vi "SERIAL_Open.vi"(7 "Serial Port (MXP)":T1=enum."MXP TTL", 9 "Reconnect":bool, 10 "Update Rate (4Hz-60Hz)":u8=50, 11 "Nav6Mode (ProcessedData)":T2) -> (0 "error out":errorcluster, 1 "Opened":bool, 3 "navX Ref":T3={"SerialPortRef"={"DevStatus"={"status"=FALSE, "code"=0, "source"=""}, "Serial Port Name"=""}, "Board Information"={"WhoAmI (50 | 0x32)"=0, "Board Revision"=0, "Firmware Major Version"=0, "Firmware Minor Version"=0, "NAVX_BOARD_CAPABILITY"={"OMNIMOUNT"=FALSE, "YAW_RESET"=FALSE, "VEL_AND_DISP"=FALSE}, "NAVX_BOARD_YAW_AXIS"={"BOARD_YAW_AXIS_UP"=FALSE, "BOARD_YAW_AXIS"=0}}, "Status"={"Update Rate Hz"=0, "Accelerometer Full-Scale Range"=0, "Gyro Full-Scale Range"=0, "NAVX_OP_STATUS"=0, "NAVX_CAL_STATUS"=0, "NAVX_SELFTEST_STATUS"=0, "NAVX_SENSOR_STATUS"={"MOVING"=FALSE, "YAW_STABLE"=FALSE, "MAG_DISTURBANCE"=FALSE, "ALTITUDE_VALID"=FALSE, "SEALEVEL_PRESS_SET"=FALSE, "FUSED_HEADING_VALID"=FALSE}}, "Offsets"={"Yaw"=0.0, "Quat W"=0.0, "Quat X"=0.0, "Quat Y"=0.0, "Quat Z"=0.0}, "Update Rate (4Hz-60Hz)"=50, "Nav6Mode (YPR)"=enum."RawSensorData", "refnum name"="", "error"={"status"=FALSE, "code"=0, "source"=""}, "Loop VI Refnum"=refnum, "Serial Port"=enum."Onboard RS-232"} {"Status"."NAVX_OP_STATUS" items=["INITIALIZING", "SELFTEST_IN_PROGRESS", "ERROR", "IMU_AUTOCAL_IN_PROGRESS", "NORMAL"]; "Status"."NAVX_CAL_STATUS" items=["IMU_CAL_STATE_MASK"=3, "IMU_CAL_INPROGRESS"=0, "IMU_CAL_ACCUMULATE"=1, "IMU_CAL_COMPLETE"=2, "MAG_CAL_COMPLETE"=4, "BARO_CAL_COMPLETE"=8]})   [LabVIEW 2014, in "navX-MXP IMU.lvlib"]
uses:
  navX-MXP IMU.lvlib
  TypeDefs/navX Serial DevRef.ctl
  <vilib>/Rock Robotics/WPI/SerialPort/WPI_SerialPortRef.ctl
  COMMON/TypeDefs/Data TypeDefs/navX Board Information.ctl
  COMMON/TypeDefs/Value TypeDefs/navX NAVX_BOARD_CAPABILITY.ctl
  COMMON/TypeDefs/Value TypeDefs/navX NAVX_BOARD_YAW_AXIS.ctl
  COMMON/TypeDefs/Data TypeDefs/navX Status Data.ctl
  COMMON/TypeDefs/Value TypeDefs/navX NAVX_OP_STATUS.ctl
  COMMON/TypeDefs/Value TypeDefs/navX NAVX_CAL_STATUS.ctl
  COMMON/TypeDefs/Value TypeDefs/navX NAVX_SENSOR_STATUS.ctl
  TypeDefs/navX Serial Mode.ctl
  NI WPI/WPI_SerialPort_USB.ctl
  <vilib>/Rock Robotics/SystemInterfaces/Utilities/FPGA_UtilitiesRead LocalTime.vi
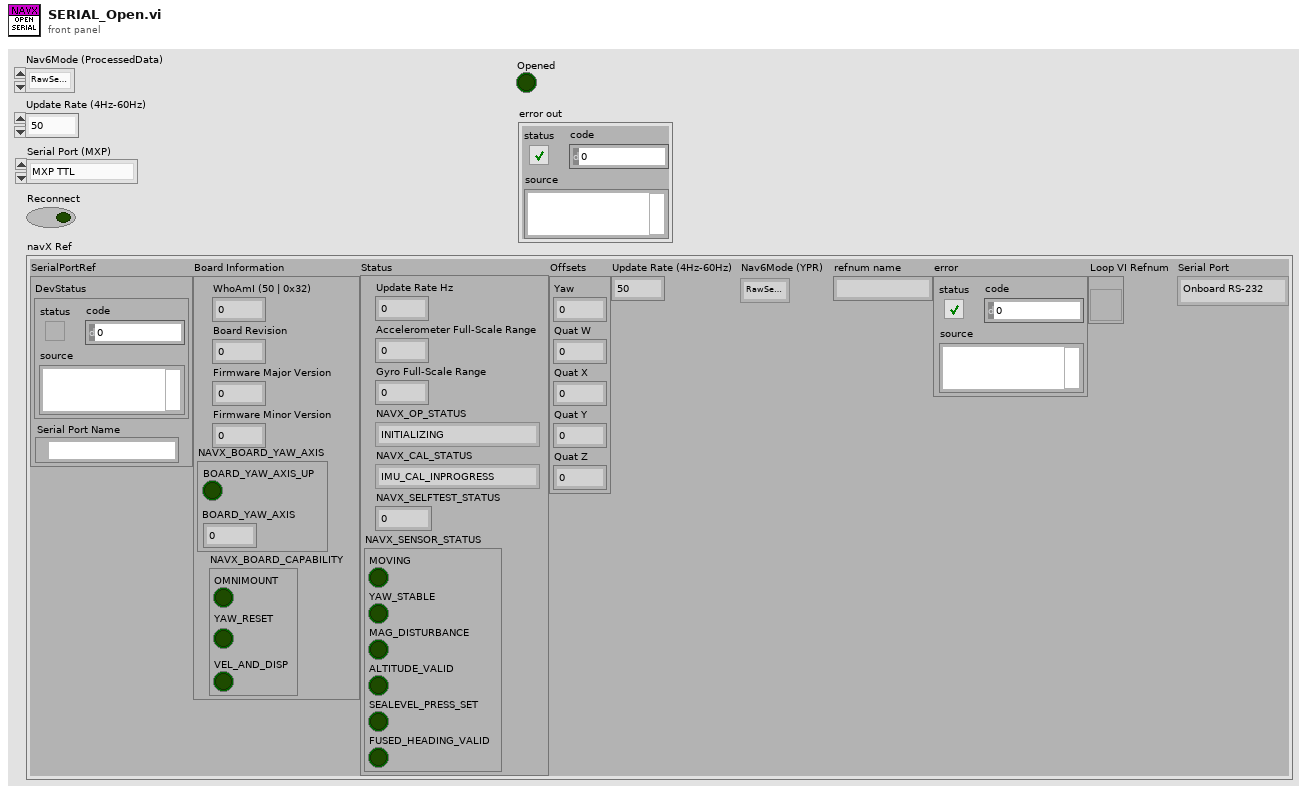
[diagram p1: front panel]
types:
  T1 = typedef "navX-MXP IMU.lvlib/WPI_SerialPort_USB.ctl" = enum16{"Onboard RS-232", "MXP TTL", "USB"}
  T2 = typedef "navX-MXP IMU.lvlib/navX Serial Mode.ctl" = enum16{"RawSensorData", "ProcessedData"}
  T3 = typedef "navX-MXP IMU.lvlib/navX Serial DevRef.ctl" = cluster{"SerialPortRef":T4, "Board Information":T5, "Status":T8, "Offsets":cluster{"Yaw":dbl, "Quat W":dbl, "Quat X":dbl, "Quat Y":dbl, "Quat Z":dbl}, "Update Rate (4Hz-60Hz)":u8, "Nav6Mode (YPR)":T2, "refnum name":string, "error":errorcluster, "Loop VI Refnum":refnum<vi>, "Serial Port":T1}
  T4 = typedef "WPI_SerialPortRef.ctl" = cluster{"DevStatus":errorcluster, "Serial Port Name":refnum<visa-resource-name>}
  T5 = typedef "navX-MXP IMU.lvlib/navX Board Information.ctl" = cluster{"WhoAmI (50 | 0x32)":u8, "Board Revision":u8, "Firmware Major Version":u8, "Firmware Minor Version":u8, "NAVX_BOARD_CAPABILITY":T6, "NAVX_BOARD_YAW_AXIS":T7}
  T6 = typedef "navX-MXP IMU.lvlib/navX NAVX_BOARD_CAPABILITY.ctl" = cluster{"OMNIMOUNT":bool, "YAW_RESET":bool, "VEL_AND_DISP":bool}
  T7 = typedef "navX-MXP IMU.lvlib/navX NAVX_BOARD_YAW_AXIS.ctl" = cluster{"BOARD_YAW_AXIS_UP":bool, "BOARD_YAW_AXIS":u8}
  T8 = typedef "navX-MXP IMU.lvlib/navX Status Data.ctl" = cluster{"Update Rate Hz":u8, "Accelerometer Full-Scale Range":u8, "Gyro Full-Scale Range":u16, "NAVX_OP_STATUS":T9, "NAVX_CAL_STATUS":T10, "NAVX_SELFTEST_STATUS":u8, "NAVX_SENSOR_STATUS":T11}
  T9 = typedef "navX-MXP IMU.lvlib/navX NAVX_OP_STATUS.ctl" = u8
  T10 = typedef "navX-MXP IMU.lvlib/navX NAVX_CAL_STATUS.ctl" = u8
  T11 = typedef "navX-MXP IMU.lvlib/navX NAVX_SENSOR_STATUS.ctl" = cluster{"MOVING":bool, "YAW_STABLE":bool, "MAG_DISTURBANCE":bool, "ALTITUDE_VALID":bool, "SEALEVEL_PRESS_SET":bool, "FUSED_HEADING_VALID":bool}
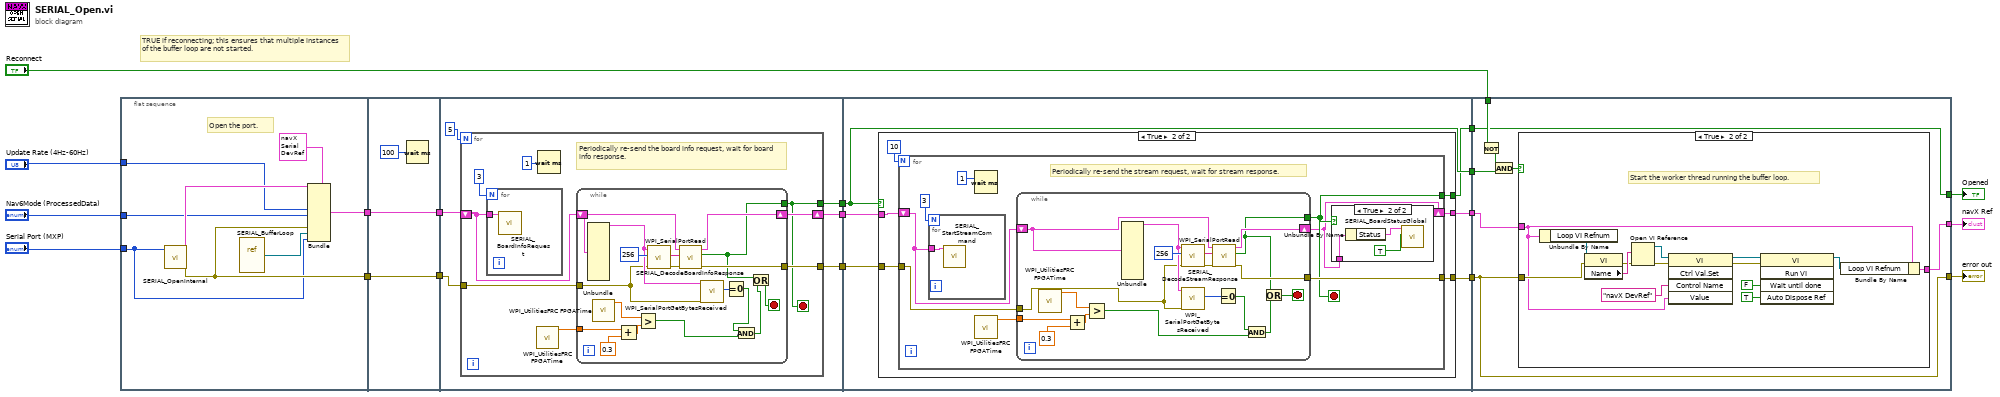
[diagram p0: block diagram]
diagram:
  # "TRUE if reconnecting; this ensures that multiple instances of the buffer loop are not started."
  n1 = flat-sequence {
    tunnel: [w26] -> w18
    tunnel: [w22] -> w7
    tunnel: "Update Rate (4Hz-60Hz)" -> [w21]
    tunnel: "Nav6Mode (ProcessedData)" -> [w20]
    tunnel: "Serial Port (MXP)" -> [w19]
    tunnel: w18 -> [w27]
    tunnel: [w28] -> w8
    tunnel: w7 -> [w28]
    tunnel: [w27] -> w6
    tunnel: [w30] -> w15
    tunnel: [w35] -> w12
    tunnel: [w34] -> w10
    tunnel: w8 -> [w31]
    tunnel: w6 -> [w33]
    tunnel: w15 -> [w64]
    tunnel: [w63] -> w14
    tunnel: [w67] -> w13
    tunnel: w12 -> [w66]
    tunnel: [w65] -> w11
    tunnel: w10 -> [w68]
    tunnel: [w68] -> w9
    tunnel: [w108] -> w1
    tunnel: [w115] -> w17
    tunnel: [w114] -> w16
    tunnel: w14 -> [w115]
    tunnel: w13 -> [w108]
    tunnel: w11 -> [w113]
    tunnel: w9 -> [w112]
    tunnel: "Reconnect" -> [w111]
    frame #0 {
      # "Open the port."
      n2 = call "SERIAL_OpenInternal.vi"("Serial Port (MXP)"=w19) -> ("error out"=w22:errorcluster, "SerialPortRef"=w23:T4)  [unwired: 8 in, 1 out]
      n3 = vi-ref "SERIAL_BufferLoop.vi"() -> (w25:refnum<vi>)
      n4 = Bundle(cluster=T3 {"SerialPortRef"={"DevStatus"={"status"=FALSE, "code"=0, "source"=""}, "Serial Port Name"=""}, "Board Information"={"WhoAmI (50 | 0x32)"=0, "Board Revision"=0, "Firmware Major Version"=0, "Firmware Minor Version"=0, "NAVX_BOARD_CAPABILITY"={"OMNIMOUNT"=FALSE, "YAW_RESET"=FALSE, "VEL_AND_DISP"=FALSE}, "NAVX_BOARD_YAW_AXIS"={"BOARD_YAW_AXIS_UP"=FALSE, "BOARD_YAW_AXIS"=0}}, "Status"={"Update Rate Hz"=0, "Accelerometer Full-Scale Range"=0, "Gyro Full-Scale Range"=0, "NAVX_OP_STATUS"=0, "NAVX_CAL_STATUS"=0, "NAVX_SELFTEST_STATUS"=0, "NAVX_SENSOR_STATUS"={"MOVING"=FALSE, "YAW_STABLE"=FALSE, "MAG_DISTURBANCE"=FALSE, "ALTITUDE_VALID"=FALSE, "SEALEVEL_PRESS_SET"=FALSE, "FUSED_HEADING_VALID"=FALSE}}, "Offsets"={"Yaw"=0.0, "Quat W"=0.0, "Quat X"=0.0, "Quat Y"=0.0, "Quat Z"=0.0}, "Update Rate (4Hz-60Hz)"=50, "Nav6Mode (YPR)"=enum."RawSensorData", "refnum name"="", "error"={"status"=FALSE, "code"=0, "source"=""}, "Loop VI Refnum"=refnum, "Serial Port"=enum."Onboard RS-232"} ("navX Ref Object"), "SerialPortRef"=w23, "Update Rate (4Hz-60Hz)"=w21, "Nav6Mode (YPR)"=w20, "error"=w22, "Loop VI Refnum"=w25, "Serial Port"=w19) -> (w26:T3)  [unwired: 4 in]
    }
    frame #1 {
      n5 = Wait (ms)(milliseconds to wait=u32 100) -> ()  [unwired: 1 out]
    }
    frame #2 {
      n6 = for {
        N: 5 -> [_]
        tunnel: [w42] -> w30
        tunnel: [w41] -> w34
        shift-right: [w43] -> w35
        shift-left: w33 -> [w39]
        tunnel: w31 -> [w38]
        stop <- w41 stop-if-true
        # "Periodically re-send the board info request, wait for board info response."
        n7 = for {
          N: 3 -> [_]
          tunnel: w39 -> [w44]
          n8 = call "SERIAL_BoardInfoRequest.vi"("navX Ref"=w44) -> ()  [unwired: 10 in, 1 out]
        }
        n9 = call <vilib>:"WPI_UtilitiesFRC FPGATime.vi"() -> ("FPGA Time"=w37:dbl)  [unwired: 10 in, 1 out]
        n10 = Wait (ms)(milliseconds to wait=u32 1) -> ()  [unwired: 1 out]
        n11 = while {
          tunnel: [w61] -> w42
          tunnel: [w55] -> w41
          shift-right: [w62] -> w43
          shift-left: w39 -> [w60]
          tunnel: w38 -> [w53]
          tunnel: w37 -> [w49]
          stop <- w54 stop-if-true
          n12 = Unbundle(w60) -> ("SerialPortRef"=w56:T4)  [unwired: 9 out]
          n13 = call <vilib>:"WPI_UtilitiesFRC FPGATime.vi"() -> ("FPGA Time"=w52:dbl)  [unwired: 10 in, 1 out]
          n14 = Add(x=w49, y=0.3) -> (x+y=w51:dbl)
          n15 = Greater?(x=w52, y=w51) -> (0:w48:bool)
          n16 = call <vilib>:"WPI_SerialPortRead.vi"("error in (no error)"=w53, "Num Bytes to Read"=u32 256, "SerialPortRef"=w56) -> ("error out"=w58:errorcluster, "Buffer"=w45:string)  [unwired: 6 in, 1 out]
          n17 = call "SERIAL_DecodeBoardInfoResponse.vi"("error in"=w58, "Buffer"=w45, "navX DevRef"=w60) -> ("error out"=w61:errorcluster, "Valid?"=w55:bool, "navX DevRef"=w62:T3)  [unwired: 6 in]
          n18 = call <vilib>:"WPI_SerialPortGetBytesReceived.vi"("error in (no error)"=w53, "SerialPortRef"=w56) -> ("Bytes at Port"=w57:u32)  [unwired: 7 in, 2 out]
          n19 = Equal To 0?(x=w57) -> (x = 0?=w47:bool)
          n20 = And(x=w47, y=w48) -> (x .and. y?=w46:bool)
          n21 = Or(x=w55, y=w46) -> (x .or. y?=w54:bool)
        }
      }
    }
    frame #3 {
      n22 = case shown="True" w68 {
        selector: w68 -> [w71 _]
        tunnel: [w71 w76] -> w67
        tunnel: w66 -> [w70 w75]
        tunnel: [w70 w74] -> w65
        tunnel: w64 -> [w69 w73]
        tunnel: [w69 w72] -> w63
        frame False {
        }
        frame True {
          n23 = for {
            N: 10 -> [_]
            tunnel: [w85] -> w72
            tunnel: [w80] -> w76
            shift-right: [w79] -> w74
            shift-left: w75 -> [w84]
            tunnel: w73 -> [w82]
            stop <- w80 stop-if-true
            # "Periodically re-send the stream request, wait for stream response."
            n24 = for {
              N: 3 -> [_]
              tunnel: w84 -> [w89]
              n25 = call "SERIAL_StartStreamCommand.vi"("navX Ref"=w89) -> ()  [unwired: 9 in, 2 out]
            }
            n26 = Wait (ms)(milliseconds to wait=u32 1) -> ()  [unwired: 1 out]
            n27 = call <vilib>:"WPI_UtilitiesFRC FPGATime.vi"() -> ("FPGA Time"=w83:dbl)  [unwired: 10 in, 1 out]
            n28 = while {
              tunnel: [w106] -> w85
              tunnel: [w100] -> w80
              shift-right: [w107] -> w79
              shift-left: w84 -> [w99]
              tunnel: w83 -> [w96]
              tunnel: w82 -> [w90]
              stop <- w98 stop-if-true
              n29 = call <vilib>:"WPI_UtilitiesFRC FPGATime.vi"() -> ("FPGA Time"=w94:dbl)  [unwired: 10 in, 1 out]
              n30 = Add(x=w96, y=0.3) -> (x+y=w95:dbl)
              n31 = Greater?(x=w94, y=w95) -> (0:w91:bool)
              n32 = Unbundle(w99) -> ("SerialPortRef"=w102:T4)  [unwired: 9 out]
              n33 = call <vilib>:"WPI_SerialPortRead.vi"("error in (no error)"=w90, "Num Bytes to Read"=u32 256, "SerialPortRef"=w102) -> ("error out"=w104:errorcluster, "Buffer"=w103:string)  [unwired: 6 in, 1 out]
              n34 = call <vilib>:"WPI_SerialPortGetBytesReceived.vi"("error in (no error)"=w90, "SerialPortRef"=w102) -> ("Bytes at Port"=w101:u32)  [unwired: 7 in, 2 out]
              n35 = call "SERIAL_DecodeStreamResponse.vi"("error in"=w104, "Buffer"=w103, "navX DevRef"=w99) -> ("error out"=w106:errorcluster, "Valid"=w100:bool, "navX DevRef"=w107:T3)  [unwired: 6 in]
              n36 = Equal To 0?(x=w101) -> (x = 0?=w93:bool)
              n37 = And(x=w93, y=w91) -> (x .and. y?=w92:bool)
              n38 = Or(x=w100, y=w92) -> (x .or. y?=w98:bool)
            }
            n39 = case shown="True" w80 {
              tunnel: w79 -> [_ w88]
              frame False {
              }
              frame True {
                n40 = Unbundle By Name(w88) -> ("Status"=w87:T8)
                n41 = call "SERIAL_BoardStatusGlobal.vi"("Set"=TRUE, "Status"=w87) -> ()  [unwired: 8 in, 2 out]
              }
            }
          }
        }
      }
    }
    frame #4 {
      n42 = Not(x=w111) -> (.not. x?=w110:bool)
      n43 = And(x=w110, y=w112) -> (x .and. y?=w109:bool)
      n44 = case shown="True" w109 {
        tunnel: w115 -> [_ w127]
        tunnel: [w116 w123] -> w114
        tunnel: w113 -> [w116 w117]
        frame False {
        }
        frame True {
          # "Start the worker thread running the buffer loop."
          n45 = Unbundle By Name(w117) -> ("Loop VI Refnum"=w130:refnum<vi>)
          n46 = property class="VI"(reference=w130, error in=w127) -> (error out=w128:errorcluster, "Name"=w129:string)  [unwired: 1 out]
          n47 = Open VI Reference(vi path=w129, error in (no error)=w128) -> (vi reference=w122:refnum<vi>, error out=w119:errorcluster)  [unwired: 4 in]
          n48 = invoke class="VI" method="Ctrl Val.Set"(reference=w122, error in=w119, "Control Name"="navX DevRef", "Value"=w117) -> (reference out=w120:refnum<vi>, error out=w118:errorcluster)  [unwired: 1 in, 3 out]
          n49 = invoke class="VI" method="Run VI"(reference=w120, error in=w118, "Wait until done"=FALSE ("Wait Until Done"), "Auto Dispose Ref"=TRUE ("Auto Dispose Reference")) -> (reference out=w124:refnum<vi>)  [unwired: 1 in, 4 out]
          n50 = Bundle By Name(cluster=w117, "Loop VI Refnum"=w124) -> (w123:T3)
        }
      }
    }
  }
  "error out" <- w17
  "navX Ref" <- w16
  "Opened" <- w1
